vi "LV Timestamp to Unix Epoch.vi"(10 "LV Timestamp (UTC)":timestamp) -> (2 "Unix Timestamp":u64)   [LabVIEW 2022 SP3, in "hse-misc.lvlib"]
doc: "Convert a LabView Timestamp (UTC Timezone) to a Unix Epoch Timestamp (C time_t).\n\n____\nHAMPEL SOFTWARE ENGINEERING v3.8.0 (2023-12-18 14:41)"
uses:
  hse-misc.lvlib
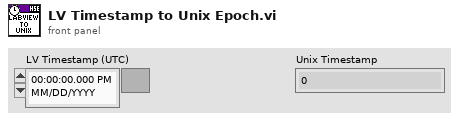
[diagram p1: front panel]
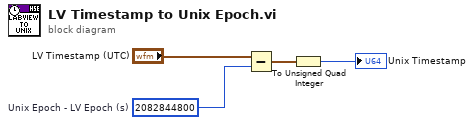
[diagram p0: block diagram]
diagram:
  w4 = u64 2082844800  # Unix Epoch - LV Epoch (s)
  n1 = Subtract(x="LV Timestamp (UTC)", y=w4) -> (x-y=w2:timestamp)
  n2 = To Unsigned Quad Integer(1:w2) -> (0:→"Unix Timestamp":u64)
